vi "Access Task From Map.vi"(8 "error in (no error)":errorcluster, 10 "ID":i64, 11 "Composite Map Task in":refnum<class "Composite Map Task.lvclass">) -> (0 "error out":errorcluster, 2 "Task Out":refnum<class "Task Ancestor.lvclass">, 3 "Composite Map Task out":refnum<class "Composite Map Task.lvclass">)   [LabVIEW 2022 SP3, in "Composite Map Task.lvclass"]
uses:
  Composite Map Task.lvclass
  Task Ancestor/Task Ancestor.lvclass
  Composite Map Task.lvclass/Composite Map Task.ctl
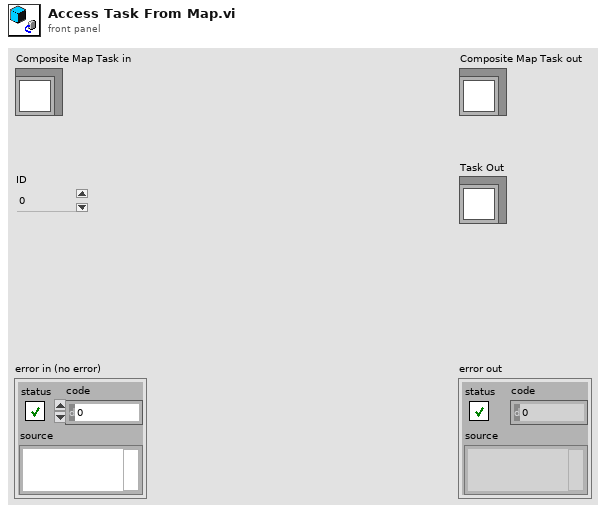
[diagram p1: front panel]
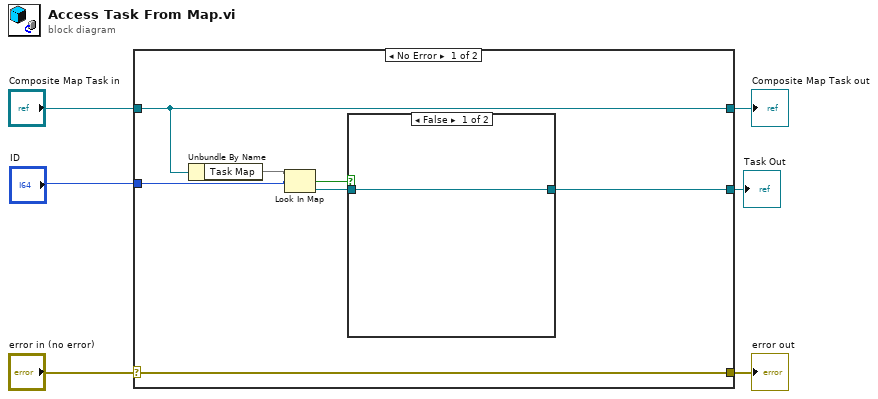
[diagram p0: block diagram]
diagram:
  n1 = case shown="No Error" "error in (no error)" {
    selector: "error in (no error)" -> [w13 w16]
    tunnel: [w13 w16] -> w5
    tunnel: [w12 w15] -> w3
    tunnel: "Composite Map Task in" -> [w12 w15]
    tunnel: "ID" -> [w10 _]
    tunnel: [w7 _] -> w1
    frame No Error {
      n2 = Unbundle By Name(w12) -> ("Task Map"=w11:map{i64, refnum<class "Task Ancestor.lvclass">})
      n3 = Look In Map(map=w11, key=w10) -> (key not found?=w9:bool, value=w8:refnum<class "Task Ancestor.lvclass">)  [unwired: 1 in]
      n4 = case shown="False" w9 {
        tunnel: w8 -> [w14 _]
        tunnel: [w14 _] -> w7
        frame False {
        }
        frame True {
        }
      }
    }
    frame Error {
    }
  }
  "error out" <- w5
  "Composite Map Task out" <- w3
  "Task Out" <- w1
